vi "DownloadCode.vi"(5 "Local Version":T1, 6 "address":string, 7 "Local Runtime":path, 8 "error in":errorcluster, 9 "port":u16=9090, 10 "Message Box":refnum<vi>, 11 "Python Source":path) -> (0 "error out":errorcluster)   [LabVIEW 2014, in "Raspberry Pi Compatible Compiler for LabVIEW.lvlib"]
uses:
  RasPi_Services/MessageBox/MessageBox.lvclass
  RasPi_Services/Download/RuntimeVersion.ctl
  Raspberry Pi Compatible Compiler for LabVIEW.lvlib
  RasPi_Services/Websocket/Websocket.lvlib
  RasPi_Services/Download/RasPiDownloader.lvlib
  Messaging/SimpleMessaging.lvlib
panel:
  in  "state variables":T2
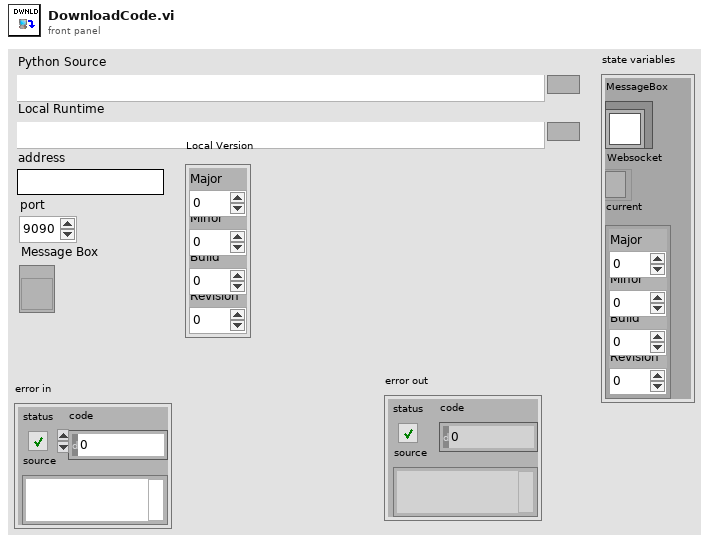
[diagram p1: front panel]
types:
  T1 = typedef "Raspberry Pi Compatible Compiler for LabVIEW.lvlib/RasPiDownloader.lvlib/RuntimeVersion.ctl" = cluster{"Major":i32, "Minor":i32, "Build":i32, "Revision":i32}
  T2 = cluster{"MessageBox":refnum<class "MessageBox.lvclass">, "Websocket":refnum<k5>, "current":T1}
  T3 = typedef "Raspberry Pi Compatible Compiler for LabVIEW.lvlib/SimpleMessaging.lvlib/MessageQueueTD.ctl" = refnum<queue>
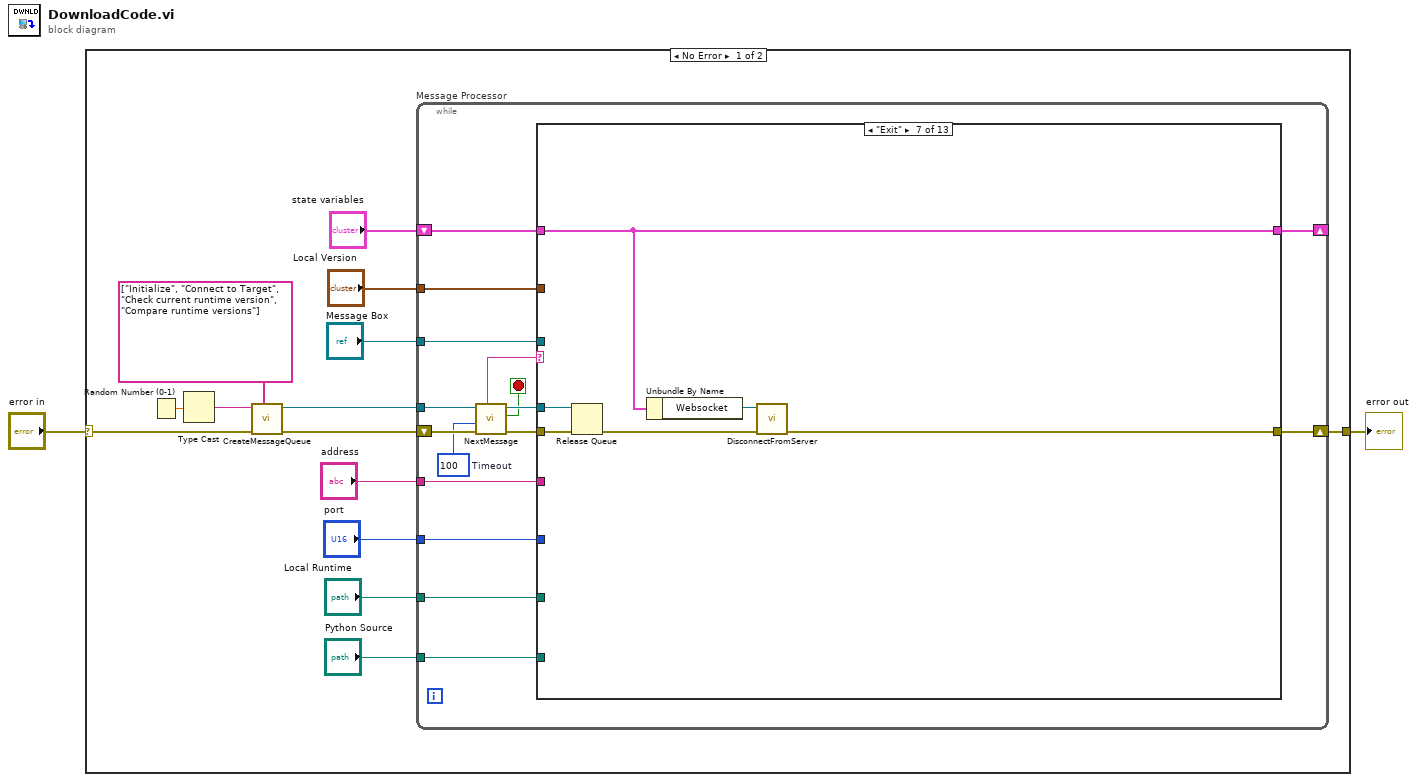
[diagram p0: block diagram]
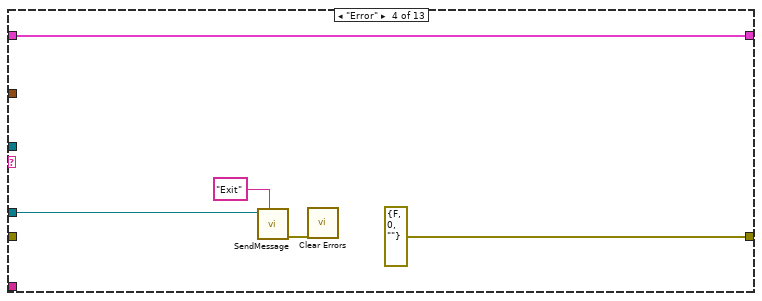
[diagram p5: hidden frame]
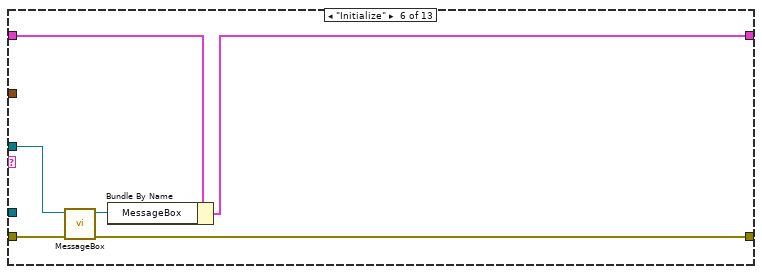
[diagram p7: hidden frame]
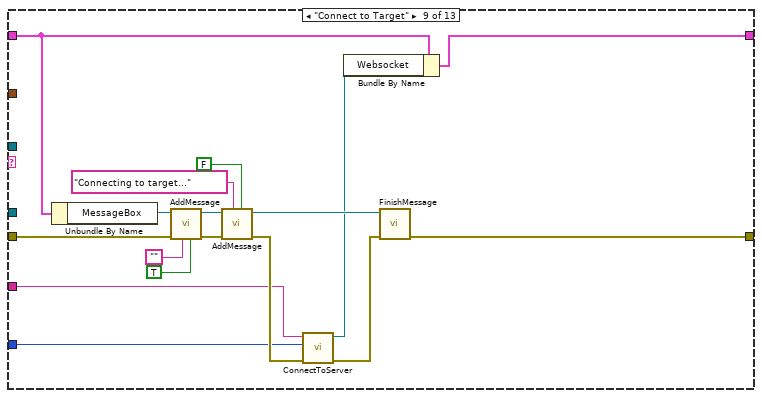
[diagram p9: hidden frame]
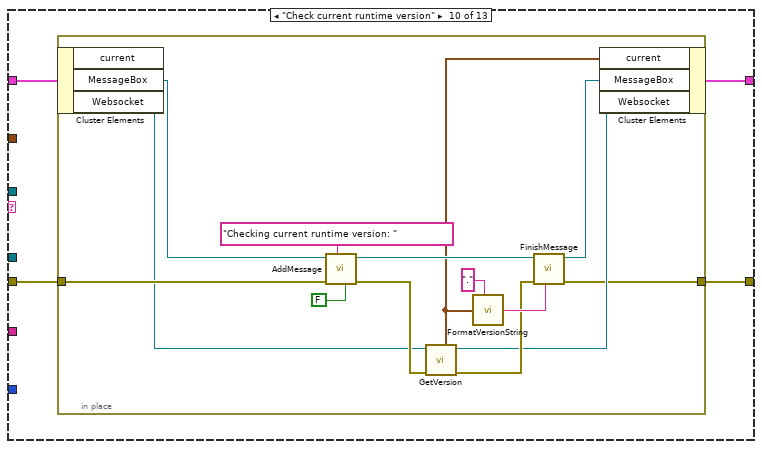
[diagram p10: hidden frame]
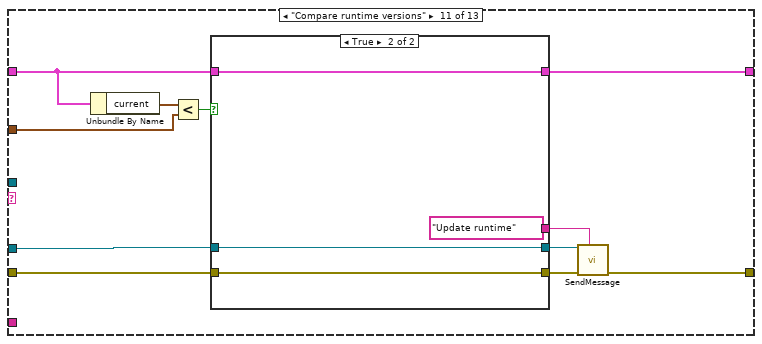
[diagram p11: hidden frame]
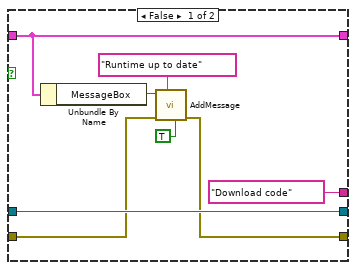
[diagram p12: hidden frame]
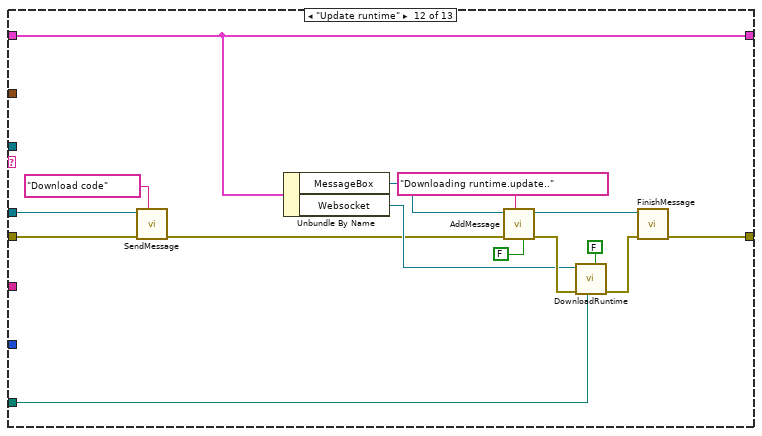
[diagram p13: hidden frame]
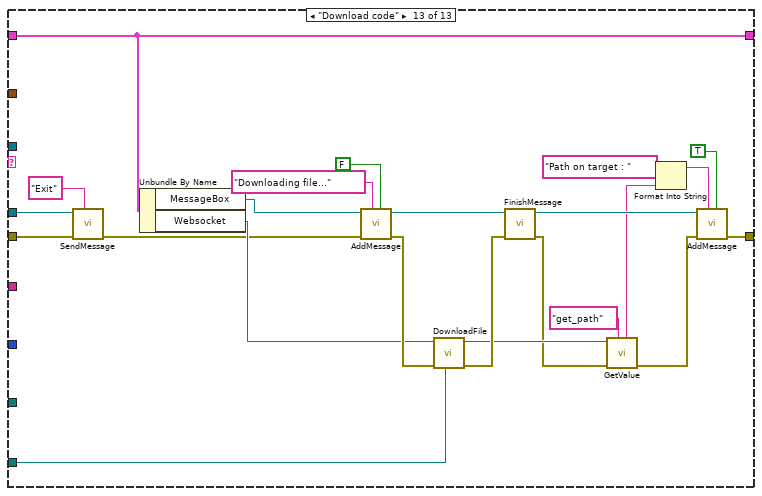
[diagram p14: hidden frame]
diagram:
  n1 = case shown="No Error" "error in" {
    selector: "error in" -> [w3 w156]
    tunnel: [w5 w156] -> w2
    frame No Error {
      n2 = Random Number (0-1)() -> (number: 0 to 1=w13:dbl)
      n3 = Type Cast(x=w13) -> (*(type *) &x=w14:string)  [unwired: 1 in]
      n4 = call "CreateMessageQueue.vi"("initial message names"=string[] ["Initialize", "Connect to Target", "Check current runtime version", "Compare runtime versions"], "error in"=w3, "message queue name"=w14) -> ("error out"=w4:errorcluster, "message queue out"=w15:T3)  [unwired: 4 in, 1 out]
      n5 = while "Message Processor" {
        shift-left: w4 -> [w27]
        shift-right: [w30] -> w5
        tunnel: w15 -> [w28]
        shift-left: "state variables" -> [w32]
        shift-right: [w31] -> _
        tunnel: "address" -> [w24]
        tunnel: "port" -> [w23]
        tunnel: "Message Box" -> [w22]
        tunnel: "Local Version" -> [w21]
        tunnel: "Local Runtime" -> [w20]
        tunnel: "Python Source" -> [w19]
        stop <- w17 stop-if-true
        w25 = 100  # Timeout
        n6 = call "NextMessage.vi"("error in"=w27, "timeout in ms (-1)"=w25, "message queue in"=w28) -> ("error out"=w26:errorcluster, "exit"=w17:bool, "message queue out"=w29:T3, "Name"=w18:string)  [unwired: 1 in, 2 out]
        n7 = case shown="\"Exit\"" w18 {
          tunnel: [w34 w36 w38 w43 w45 w47 w55 w59 w67 w79 w99 w124 w138] -> w31
          tunnel: w32 -> [w34 w36 w38 w43 w45 w49 w55 w59 w66 w80 w100 w124 w138]
          tunnel: w29 -> [_ _ _ w41 _ _ w56 _ _ _ w102 w122 w135]
          tunnel: w26 -> [w33 w35 w37 _ w44 w51 w57 w58 w63 w77 w101 w123 w136]
          tunnel: [w33 w35 w37 errorcluster {"status"=FALSE, "code"=0, "source"=""} ("error out") w44 w46 w52 w58 w72 w78 w96 w132 w139] -> w30
          tunnel: w24 -> [_ _ _ _ _ _ _ _ w69 _ _ _ _]
          tunnel: w23 -> [_ _ _ _ _ _ _ _ w70 _ _ _ _]
          tunnel: w22 -> [_ _ _ _ _ w50 _ _ _ _ _ _ _]
          tunnel: w21 -> [_ _ _ _ _ _ _ _ _ _ w104 _ _]
          tunnel: w20 -> [_ _ _ _ _ _ _ _ _ _ _ w118 _]
          tunnel: w19 -> [_ _ _ _ _ _ _ _ _ _ _ _ w140]
          frame "---------- Framework Operations ----------" {
          }
          frame "", "Idle" {
          }
          frame Default {
          }
          frame "Error" {
            n8 = call "SendMessage.vi"("Name"="Exit", "message queue in"=w41) -> ("error out"=w39:errorcluster)  [unwired: 5 in, 2 out]
            n9 = call <vilib>:"Clear Errors.vi"("error in (no error)"=w39) -> ()  [unwired: 5 in, 2 out]
          }
          frame "---------- Generic Operations ----------" {
          }
          frame "Initialize" {
            n10 = call "MessageBox.vi"("error in"=w51, "Message Box"=w50) -> ("error out"=w46:errorcluster, "MessageBox out"=w48:refnum<class "MessageBox.lvclass">)  [unwired: 8 in]
            n11 = Bundle By Name(cluster=w49, "MessageBox"=w48) -> (w47:T2)
          }
          frame "Exit" {
            n12 = Release Queue(queue=w56, error in (no error)=w57) -> (error out=w54:errorcluster)  [unwired: 1 in, 2 out]
            n13 = Unbundle By Name(w55) -> ("Websocket"=w53:refnum<k5>)
            n14 = call "DisconnectFromServer.vi"("error in"=w54, "connection ID"=w53) -> ("error out"=w52:errorcluster)  [unwired: 7 in]
          }
          frame "---------- Application Operations ----------" {
          }
          frame "Connect to Target" {
            n15 = Unbundle By Name(w66) -> ("MessageBox"=w62:refnum<class "MessageBox.lvclass">)
            n16 = call "AddMessage.vi"("add newline"=TRUE, "message"="", "error in"=w63, "MessageBox in"=w62) -> ("error out"=w65:errorcluster, "MessageBox out"=w64:refnum<class "MessageBox.lvclass">)  [unwired: 4 in]
            n17 = call "AddMessage.vi"("add newline"=FALSE, "message"="Connecting to target...", "error in"=w65, "MessageBox in"=w64) -> ("error out"=w75:errorcluster, "MessageBox out"=w74:refnum<class "MessageBox.lvclass">)  [unwired: 4 in]
            n18 = call "ConnectToServer.vi"("error in"=w75, "port"=w70, "address"=w69) -> ("error out"=w73:errorcluster, "connection ID"=w68:refnum<k5>)  [unwired: 5 in, 2 out]
            n19 = Bundle By Name(cluster=w66, "Websocket"=w68) -> (w67:T2)
            n20 = call "FinishMessage.vi"("error in"=w73, "MessageBox in"=w74) -> ("error out"=w72:errorcluster)  [unwired: 6 in, 1 out]
          }
          frame "Check current runtime version" {
            n21 = in-place {
              in-place-border: [w85] -> w78
              in-place-border: w77 -> [w84]
              n22 = in-place-cluster #1(w80) -> ("MessageBox"=w83:refnum<class "MessageBox.lvclass">, "Websocket"=w82:refnum<k5>)  [unwired: 1 out]
              n23 = call "AddMessage.vi"("add newline"=FALSE, "message"="Checking current runtime version: ", "error in"=w84, "MessageBox in"=w83) -> ("error out"=w90:errorcluster, "MessageBox out"=w92:refnum<class "MessageBox.lvclass">)  [unwired: 4 in]
              n24 = call "GetVersion.vi"("error in"=w90, "connection ID"=w82) -> ("error out"=w93:errorcluster, "connection ID out"=w86:refnum<k5>, "Version"=w81:T1)  [unwired: 5 in]
              n25 = call "FormatVersionString.vi"("Version"=w81, "delimiter"=".") -> ("Version string"=w94:string)  [unwired: 1 in]
              n26 = call "FinishMessage.vi"("no error"=w94, "error in"=w93, "MessageBox in"=w92) -> ("error out"=w85:errorcluster, "MessageBox out"=w87:refnum<class "MessageBox.lvclass">)  [unwired: 5 in]
              n27 = in-place-cluster #1("current"=w81, "MessageBox"=w87, "Websocket"=w86) -> (w79:T2)
            }
          }
          frame "Compare runtime versions" {
            n28 = Unbundle By Name(w100) -> ("current"=w105:T1)
            n29 = Less?(x=w105, y=w104) -> (x < y?=w103:bool)
            n30 = case shown="True" w103 {
              tunnel: w102 -> [w109 w116]
              tunnel: w101 -> [w108 w115]
              tunnel: w100 -> [w110 w117]
              tunnel: [w110 w117] -> w99
              tunnel: [w107 w115] -> w97
              tunnel: [w109 w116] -> w98
              tunnel: ["Download code" "Update runtime"] -> w95
              frame False {
                n31 = Unbundle By Name(w110) -> ("MessageBox"=w111:refnum<class "MessageBox.lvclass">)
                n32 = call "AddMessage.vi"("add newline"=TRUE, "message"="Runtime up to date", "error in"=w108, "MessageBox in"=w111) -> ("error out"=w107:errorcluster)  [unwired: 4 in, 1 out]
              }
              frame True {
              }
            }
            n33 = call "SendMessage.vi"("Name"=w95, "error in"=w97, "message queue in"=w98) -> ("error out"=w96:errorcluster)  [unwired: 4 in, 2 out]
          }
          frame "Update runtime" {
            n34 = call "SendMessage.vi"("Name"="Download code" ("message name"), "error in"=w123, "message queue in"=w122) -> ("error out"=w121:errorcluster)  [unwired: 4 in, 2 out]
            n35 = Unbundle By Name(w124) -> ("MessageBox"=w125:refnum<class "MessageBox.lvclass">, "Websocket"=w126:refnum<k5>)
            n36 = call "AddMessage.vi"("add newline"=FALSE, "message"="Downloading runtime.update..", "error in"=w121, "MessageBox in"=w125) -> ("error out"=w129:errorcluster, "MessageBox out"=w128:refnum<class "MessageBox.lvclass">)  [unwired: 4 in]
            n37 = call "DownloadRuntime.vi"("check version"=FALSE, "Path"=w118, "error in"=w129, "WebSocket connection"=w126) -> ("error out"=w127:errorcluster)  [unwired: 4 in, 1 out]
            n38 = call "FinishMessage.vi"("error in"=w127, "MessageBox in"=w128) -> ("error out"=w132:errorcluster)  [unwired: 6 in, 1 out]
          }
          frame "Download code" {
            n39 = call "SendMessage.vi"("Name"="Exit" ("message name"), "error in"=w136, "message queue in"=w135) -> ("error out"=w133:errorcluster)  [unwired: 4 in, 2 out]
            n40 = Unbundle By Name(w138) -> ("MessageBox"=w134:refnum<class "MessageBox.lvclass">, "Websocket"=w141:refnum<k5>)
            n41 = call "AddMessage.vi"("add newline"=FALSE, "message"="Downloading file...", "error in"=w133, "MessageBox in"=w134) -> ("error out"=w153:errorcluster, "MessageBox out"=w152:refnum<class "MessageBox.lvclass">)  [unwired: 4 in]
            n42 = call "DownloadFile.vi"("Path"=w140, "error in"=w153, "WebSocket connection"=w141) -> ("error out"=w151:errorcluster, "WebSocket connection out"=w150:refnum<k5>)  [unwired: 5 in]
            n43 = call "FinishMessage.vi"("error in"=w151, "MessageBox in"=w152) -> ("error out"=w148:errorcluster, "MessageBox out"=w146:refnum<class "MessageBox.lvclass">)  [unwired: 6 in]
            n44 = call "GetValue.vi"("cmd"="get_path", "error in"=w148, "connection ID"=w150) -> ("error out"=w147:errorcluster, "value"=w145:string)  [unwired: 4 in, 1 out]
            n45 = Format Into String(initial string="Path on target : ", w145) -> (resulting string=w144:string)  [unwired: 2 in, 1 out]
            n46 = call "AddMessage.vi"("add newline"=TRUE, "message"=w144, "error in"=w147, "MessageBox in"=w146) -> ("error out"=w139:errorcluster)  [unwired: 4 in, 1 out]
          }
        }
      }
    }
    frame Error {
    }
  }
  "error out" <- w2
